vi "Update UI.vi"(8 "error in (no error)":errorcluster, 10 "Message":string, 11 "MGI_Progress Bar in":refnum<class "Progress Bar.lvclass">) -> (0 "error out":errorcluster, 2 "Aborted":bool, 3 "MGI_Progress Bar out":refnum<class "Progress Bar.lvclass">)   [LabVIEW 2016, in "Progress Bar.lvclass"]
doc: "Updates the ui. It will open the UI if needed\n\nCopyright: MGI\nAuthored by: Derek Trepanier"
uses:
  <userlib>/_MGI/User Interface/Progress Bar/Progress Bar.lvclass
  <userlib>/_MGI/User Interface/Progress Bar/Progress Bar.lvclass/Progress Bar.ctl
  <userlib>/_MGI/User Interface/Progress Bar/Progress Bar Settings/Progress Bar Settings.lvclass
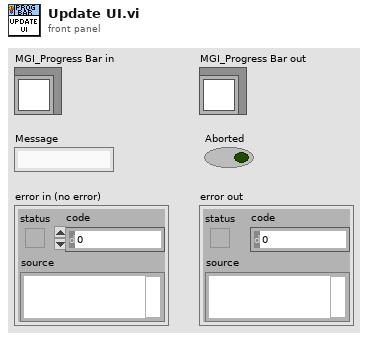
[diagram p1: front panel]
types:
  T1 = enum32{"Invalid", "Standard", "Closed", "Hidden", "Minimized", "Maximized"}
  T2 = enum32{"Invalid", "Default", "Floating", "Floating/Auto-Hide", "Modal"}
  T3 = typedef "LVRectTypeDef.ctl" = cluster{"Left":i16, "Top":i16, "Right":i16, "Bottom":i16}
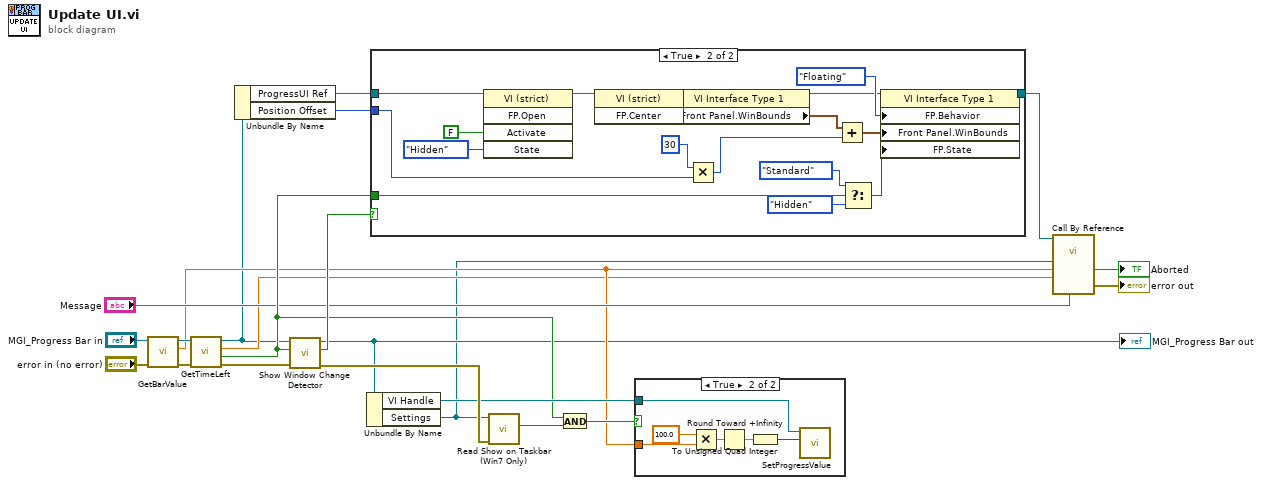
[diagram p0: block diagram]
diagram:
  n1 = call-dynamic "GetBarValue.vi"("error in (no error)"="error in (no error)", "MGI_Progress Bar in"="MGI_Progress Bar in") -> ("error out"=w21:errorcluster, "Progress Bar Value (0-100)"=w5:dbl, "MGI_Progress Bar out"=w20:refnum<class "Progress Bar.lvclass">)  [unwired: 7 in]
  n2 = call-dynamic "GetTimeLeft.vi"("error in (no error)"=w21, "MGI_Progress Bar in"=w20) -> ("error out"=w15:errorcluster, "Show Window?"=w10:bool, "Time Left"=w4:dbl, "MGI_Progress Bar out"=w3:refnum<class "Progress Bar.lvclass">)  [unwired: 6 in]
  n3 = Unbundle By Name(w3) -> ("ProgressUI Ref"=w18:refnum<vi>, "Position Offset"=w17:i16)
  n4 = call <userlib>:"Show Window Change Detector.vi"("error in (no error)"=w15, "Show Window"=w10, "Progress Bar in"=w3) -> ("error out"=w13:errorcluster, "Changed?"=w16:bool, "Progress Bar out"=w2:refnum<class "Progress Bar.lvclass">)  [unwired: 6 in]
  "MGI_Progress Bar out" <- w2
  n5 = Unbundle By Name(w2) -> ("VI Handle"=w12:refnum<k24>, "Settings"=w1:refnum<class "Progress Bar Settings.lvclass">)
  n6 = case shown="True" w16 {
    tunnel: [w23 w40] -> w9
    tunnel: w10 -> [_ w39]
    tunnel: w18 -> [w23 w36]
    tunnel: w17 -> [_ w26]
    frame False {
    }
    frame True {
      n7 = invoke class="VI (strict)" method="FP.Open"(reference=w36, "Activate"=FALSE ("Activate?"), "State"=T1."Hidden") -> (reference out=w37:refnum<vi>)  [unwired: 2 in, 4 out]
      n8 = invoke class="VI (strict)" method="FP.Center"(reference=w37) -> (reference out=w35:refnum<vi>)  [unwired: 2 in, 2 out]
      n9 = property class="VI Interface Type 1"(reference=w35) -> (reference out=w33:refnum<vi>, "Front Panel.WinBounds"=w31:T3)  [unwired: 1 in, 1 out]
      n10 = Multiply(x=i16 30 ("y"), y=w26) -> (x*y=w32:i16)
      n11 = Add(x=w31, y=w32) -> (x+y=w30:T3)
      n12 = Select(t=T1."Standard" ("State"), s=w39, f=T1."Hidden") -> (s? t:f=w25:T1)
      n13 = property class="VI Interface Type 1"(reference=w33, "FP.Behavior"=T2."Floating" ("Front Panel Window:Behavior"), "Front Panel.WinBounds"=w30, "FP.State"=w25) -> (reference out=w40:refnum<vi>)  [unwired: 1 in, 1 out]
    }
  }
  n14 = call-dynamic "Read Show on Taskbar (Win7 Only).vi"("error in (no error)"=w13, "MGI_Progress Bar Options in"=w1) -> ("Show on Taskbar (Win7 Only)"=w14:bool)  [unwired: 7 in, 2 out]
  n15 = And(x=w10, y=w14) -> (x .and. y?=w11:bool)
  n16 = case shown="True" w11 {
    tunnel: w5 -> [_ w46]
    tunnel: w12 -> [_ w42]
    frame False {
    }
    frame True {
      n17 = Multiply(x=100.0, y=w46) -> (x*y=w44:dbl)
      n18 = Round Toward +Infinity(x=w44) -> (ceil(x): smallest int >= x=w43:dbl)
      n19 = To Unsigned Quad Integer(1:w43) -> (0:w41:u64)
      n20 = call <userlib>:"SetProgressValue.vi"("current (0)"=w41, "Window Handle"=w42) -> ()  [unwired: 8 in, 2 out]
    }
  }
  n21 = call-by-ref "?"(reference=w9, "Message"="Message", "Time Remaining"=w4, "Progress Bar"=w5, "Settings"=w1) -> ("error out"=→"error out":errorcluster, "Aborted"=→"Aborted":bool)  [unwired: 7 in, 2 out]
